vi "PAQmem_ReadTableInfo.vi"(8 "error in (no error)":errorcluster, 11 "PAQ-memory in":refnum<class "PAQ-memory.lvclass">) -> (0 "error out":errorcluster, 2 "MemMap-element":T1, 3 "PAQ-memory out":refnum<class "PAQ-memory.lvclass">)   [LabVIEW 2020, in "Sgraph_lib_V1.lvlib" / "PAQ-memory.lvclass"]
uses:
  PAQ-memory.lvclass
  Common/controls/MMap_element.ctl
  PAQ-memory.lvclass/PAQ-memory.ctl
  MemMap/MemoryMap.lvclass
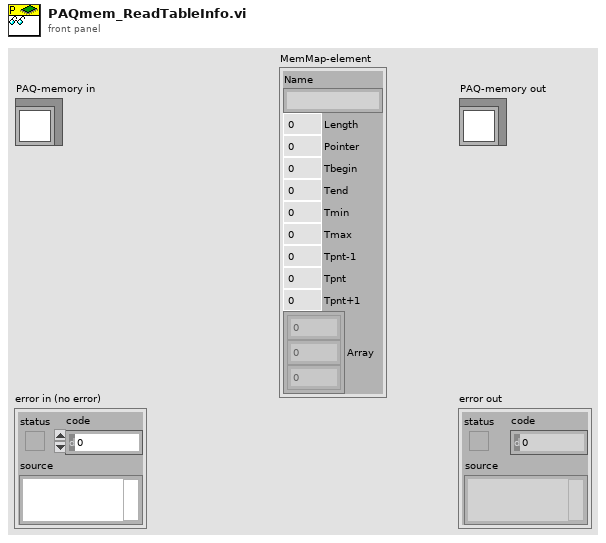
[diagram p1: front panel]
types:
  T1 = typedef "Sgraph_lib_V1.lvlib/MemoryMap.lvclass/MMap_element.ctl" = cluster{"Name":string, "Length":i32, "Pointer":i32, "Tbegin":dbl, "Tend":dbl, "Tmin":dbl, "Tmax":dbl, "Tpnt-1":dbl, "Tpnt":dbl, "Tpnt+1":dbl, "Array":dbl[]}
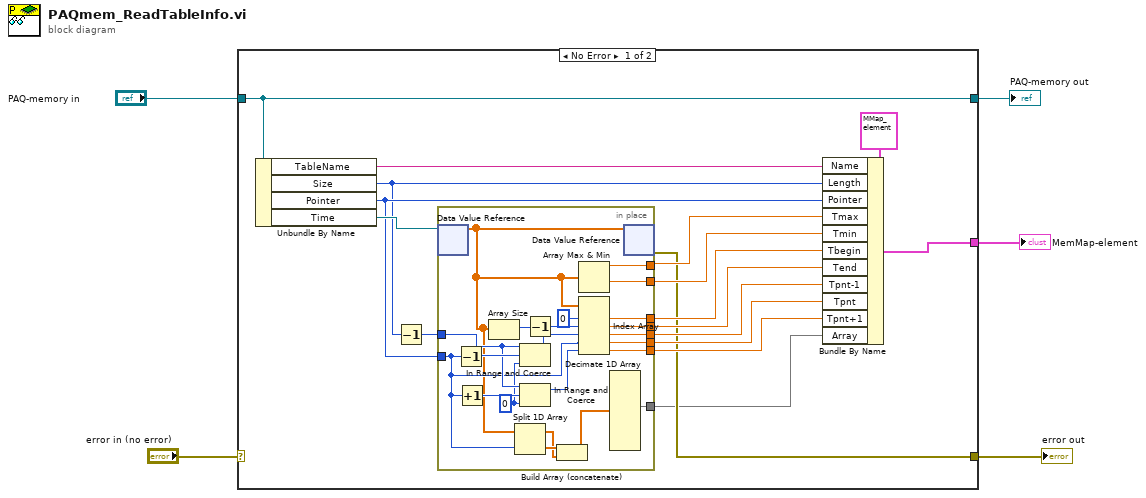
[diagram p0: block diagram]
diagram:
  n1 = case shown="No Error" "error in (no error)" {
    selector: "error in (no error)" -> [_ w45]
    tunnel: [w8 w45] -> w4
    tunnel: [w22 w46] -> w2
    tunnel: "PAQ-memory in" -> [w22 w46]
    tunnel: [w7 _] -> w1
    frame No Error {
      n2 = Unbundle By Name(w22) -> ("TableName"=w20:string, "Size"=w13:i32, "Pointer"=w14:i32, "Time"=w19:refnum<data-value>)
      n3 = Decrement(x=w13) -> (x-1=w12:i32)
      n4 = in-place {
        in-place-border: [w44] -> w18
        in-place-border: [w43] -> w17
        in-place-border: [w41] -> w16
        in-place-border: [w38] -> w15
        in-place-border: w14 -> [w27]
        in-place-border: w12 -> [w35]
        in-place-border: [w31] -> w11
        in-place-border: [w30] -> w10
        in-place-border: [w29] -> w9
        in-place-border: [w28] -> w6
        w34 = 0 ("index")
        n5 = in-place-dvr #1(w19) -> (w26:dbl[])  [unwired: 1 out]
        n6 = Decrement(x=w27) -> (x-1=w37:i32)
        n7 = Increment(x=w27) -> (x+1=w36:i32)
        n8 = Array Size(array=w26) -> (size(s)=w40:i32)
        n9 = Split 1D Array(array=w26, index=w27) -> (first subarray=w24:dbl[], second subarray=w25:dbl[])
        n10 = In Range and Coerce(upper limit=w35, x=w37, lower limit=w34) -> (coerced(x)=w33:i32)  [unwired: 1 out]
        n11 = In Range and Coerce(upper limit=w35, x=w36, lower limit=w34) -> (coerced(x)=w32:i32)  [unwired: 1 out]
        n12 = Decrement(x=w40) -> (x-1=w39:i32)
        n13 = Build Array (concatenate)(w25, w24) -> (w23:dbl[])
        n14 = Array Max & Min(array=w26) -> (max value=w44:dbl, min value=w43:dbl)  [unwired: 2 out]
        n15 = Index Array(array=w26, index #1=0 ("index"), index #2=w39, index #3=w33, index #4=w27, index #5=w32) -> (element #1=w41:dbl, element #2=w38:dbl, element #3=w31:dbl, element #4=w30:dbl, element #5=w29:dbl)
        n16 = Decimate 1D Array(w23) -> (w28:dbl[])  [unwired: 9 out]
        n17 = in-place-dvr #1(w26) -> (w8:errorcluster)  [unwired: 1 out]
      }
      n18 = Bundle By Name(cluster=T1 {"Name"="", "Length"=0, "Pointer"=0, "Tbegin"=0.0, "Tend"=0.0, "Tmin"=0.0, "Tmax"=0.0, "Tpnt-1"=0.0, "Tpnt"=0.0, "Tpnt+1"=0.0, "Array"=[]} ("MemoryInfo"), "Name"=w20, "Length"=w13, "Pointer"=w14, "Tmax"=w18, "Tmin"=w17, "Tbegin"=w16, "Tend"=w15, "Tpnt-1"=w11, "Tpnt"=w10, "Tpnt+1"=w9, "Array"=w6) -> (w7:T1)
    }
    frame Error {
    }
  }
  "error out" <- w4
  "PAQ-memory out" <- w2
  "MemMap-element" <- w1
